vi "gameover.vi"(0 "Cluster":cluster{"OK Button":bool, "String":string}={"OK Button"=FALSE, "String"="GAME OVER"}) -> ()   [LabVIEW 2014]
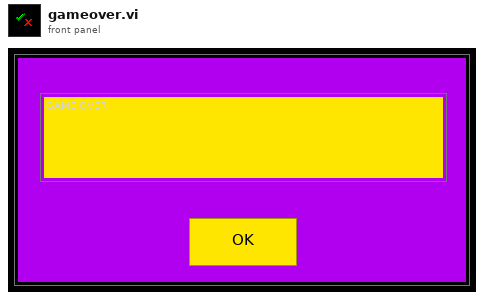
[diagram p1: front panel]
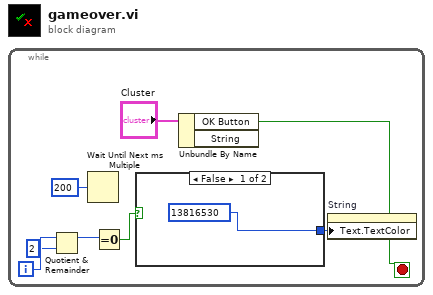
[diagram p0: block diagram]
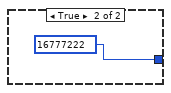
[diagram p2: hidden frame]
diagram:
  n1 = while {
    i -> [w6]
    stop <- w7 stop-if-true
    n2 = Quotient & Remainder(x=w6, y=2) -> (x-y*floor(x/y)=w4:i32)  [unwired: 1 out]
    n3 = Wait Until Next ms Multiple(millisecond multiple=u32 200) -> ()  [unwired: 1 out]
    n4 = Equal To 0?(x=w4) -> (x = 0?=w3:bool)
    n5 = case shown="False" w3 {
      tunnel: [u32 13816530 ("Text.Text Colors:Text Color") u32 16777222 ("Text.Text Colors:Text Color")] -> w2
      frame False {
      }
      frame True {
      }
    }
    n6 = Unbundle By Name("Cluster") -> ("OK Button"=w7:bool)  [unwired: 1 out]
    n7 = property on="String" class="Str"("Text.TextColor"=w2) -> ()  [unwired: 2 in, 2 out]
  }
